vi "Tool Valve decoder.vi"(0 "Force NA(F)":bool, 7 "Valve Relay code":u8 format="%08b") -> (4 "Valve LSB(0)":T1, 6 "Valve 1":T1, 8 "Valve 2":T1, 10 "Valve 3":T1, 14 "Array of valv Relay states":T1[](array[typedef]))   [LabVIEW 2011]
uses:
  Measurments Handling/Status Digitalish.ctl
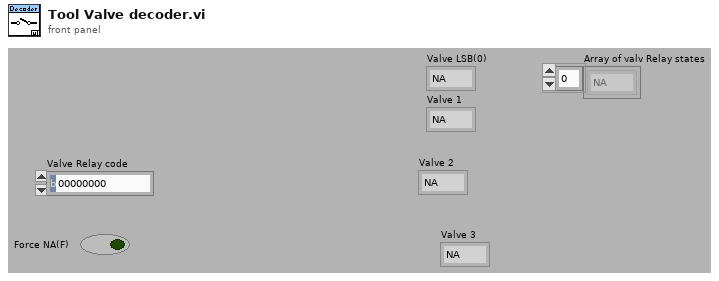
[diagram p1: front panel]
types:
  T1 = typedef "Status Digitalish.ctl" = enum16{"NA", "False", "True"}
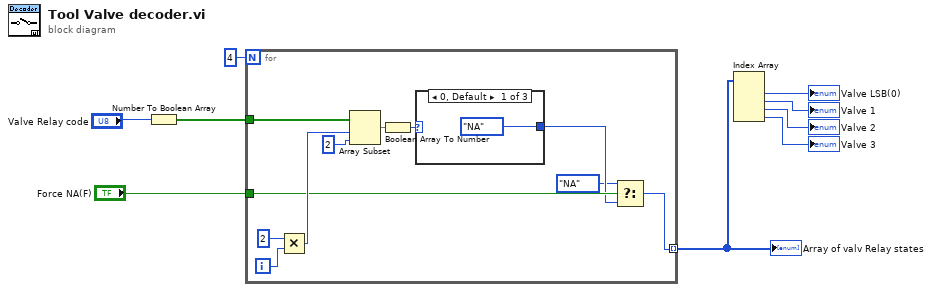
[diagram p0: block diagram]
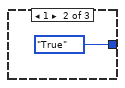
[diagram p2: hidden frame]
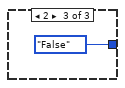
[diagram p3: hidden frame]
diagram:
  n1 = Number To Boolean Array(number="Valve Relay code") -> (Boolean array=w7:bool[])
  n2 = for {
    N: 4 -> [_]
    tunnel: w7 -> [w20]
    tunnel: [w10] -> w6 mode=indexing
    tunnel: "Force NA(F)" -> [w13]
    i -> [w19]
    n3 = Multiply(x=2, y=w19) -> (x*y=w17:i32)
    n4 = Array Subset(array=w20, index=w17, length=2) -> (w15:bool[])
    n5 = Boolean Array To Number(Boolean array=w15) -> (number=w14:u32)
    n6 = case shown="0, Default" w14 {
      tunnel: [Status_Digitalish."NA" ("Status") Status_Digitalish."True" ("Status") Status_Digitalish."False" ("Status")] -> w12
      frame 0, Default {
      }
      frame 1 {
      }
      frame 2 {
      }
    }
    n7 = Select(t=Status_Digitalish."NA", s=w13, f=w12) -> (s? t:f=w10:T1)
  }
  "Array of valv Relay states" <- w6
  n8 = Index Array(array=w6) -> (element #1=→"Valve LSB(0)":T1, element #2=→"Valve 1":T1, element #3=→"Valve 2":T1, element #4=→"Valve 3":T1)  [unwired: 4 in]
